vi "Check Device Type.vi"(8 "error in (no error)":errorcluster, 9 "Device Type Name":string, 10 "Template in":refnum<class "Template.lvclass">) -> (0 "error out":errorcluster, 1 "correct Device":bool, 2 "Template out":refnum<class "Template.lvclass">)   [LabVIEW 2011, in "Tinkerforge.lvlib" / "Template.lvclass"]
doc: "This VI is the child implementation of \"Check Device Type.vi\" and invokes the device type validation through checking the device name."
uses:
  Template.lvclass
  Device/Device.lvclass
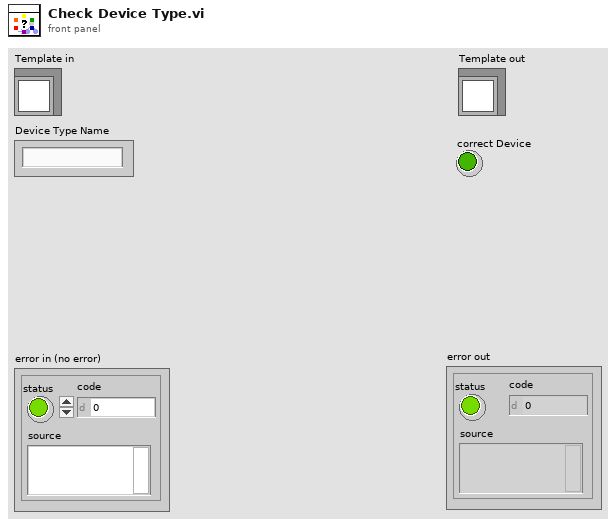
[diagram p1: front panel]
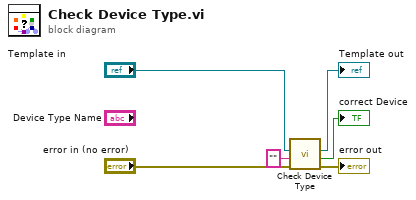
[diagram p0: block diagram]
diagram:
  n1 = call-parent "Check Device Type.vi"("error in (no error)"="error in (no error)", "Device Type Name"="", "Device in"="Template in") -> ("error out"=→"error out":errorcluster, "correct Device"=→"correct Device":bool, "Device out"=→"Template out":refnum<class "Template.lvclass">)  [unwired: 6 in]
